vi "createProjectItem.vi"(8 "error in (no error)":errorcluster, 10 "ProjectItemSelection":T1, 11 "ProjectItemFactory in":refnum<class "ProjectItemFactory.lvclass">) -> (0 "error out":errorcluster, 2 "ProjectItem":refnum<class "ProjectItem.lvclass">, 3 "ProjectItemFactory out":refnum<class "ProjectItemFactory.lvclass">)   [LabVIEW 2016, in "ProjectItemFactory.lvclass"]
uses:
  ProjectItemFactory.lvclass
  Typedefs/ProjectItemSelection.ctl
  ProjectItem/ProjectItem.lvclass
  ProjectItems/Default/Default.lvclass
  C:/LSST_TS/SystemSW/ct_tools/ProjectItem/ProjectItem.lvclass
  ProjectItems/Dependencies/Dependencies.lvclass
  ProjectItems/Folder/Folder.lvclass
  ProjectItems/Library/Library.lvclass
  ProjectItems/LVClass/LVClass.lvclass
  ProjectItems/VI/VI.lvclass
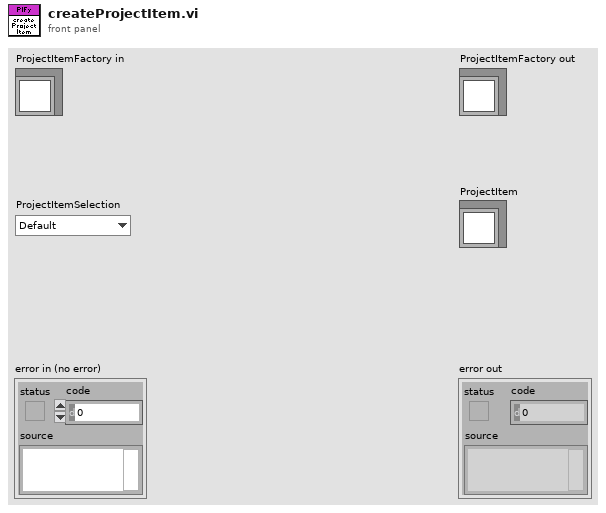
[diagram p1: front panel]
types:
  T1 = typedef "ProjectItemSelection.ctl" = enum16{"Default", "Dependencies", "Folder", "Library", "LVClass", "VI"}
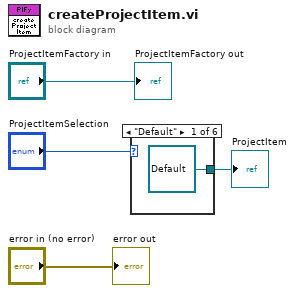
[diagram p0: block diagram]
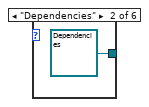
[diagram p2: hidden frame]
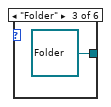
[diagram p3: hidden frame]
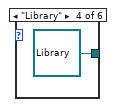
[diagram p4: hidden frame]
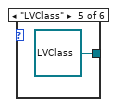
[diagram p5: hidden frame]
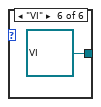
[diagram p6: hidden frame]
diagram:
  n1 = case shown="\"Default\"" "ProjectItemSelection" {
    tunnel: [refnum<class "Default.lvclass"> refnum ("Default.lvclass") refnum<class "Dependencies.lvclass"> refnum ("Dependencies.lvclass") refnum<class "Folder.lvclass"> refnum ("Folder.lvclass") refnum<class "Library.lvclass"> refnum ("Library.lvclass") refnum<class "LVClass.lvclass"> refnum ("LVClass.lvclass") refnum<class "VI.lvclass"> refnum ("VI.lvclass")] -> w2
    frame "Default" {
    }
    frame "Dependencies" {
    }
    frame "Folder" {
    }
    frame "Library" {
    }
    frame "LVClass" {
    }
    frame "VI" {
    }
  }
  "ProjectItem" <- w2
  "error out" <- "error in (no error)"
  "ProjectItemFactory out" <- "ProjectItemFactory in"
